vi "Delete Header Content Object.vi"(8 "error in (no error)":errorcluster, 11 "Header in":refnum<class "Simulated_Header.lvclass">) -> (0 "error out":errorcluster, 3 "Header out":refnum<class "Simulated_Header.lvclass">)   [LabVIEW 2018, in "Simulated_Header.lvclass"]
uses:
  Simulated_Header.lvclass
  Header Contents/Header Contents.lvclass
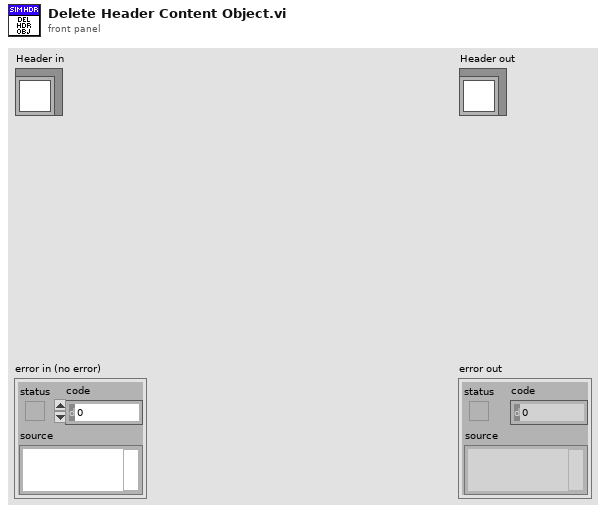
[diagram p1: front panel]
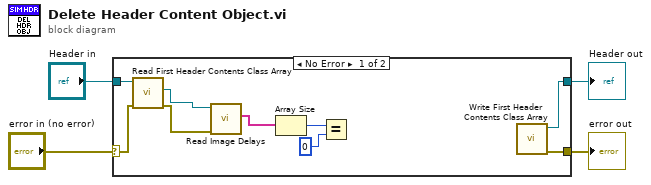
[diagram p0: block diagram]
diagram:
  n1 = case shown="No Error" "error in (no error)" {
    selector: "error in (no error)" -> [w11 w15]
    tunnel: [w12 w15] -> w3
    tunnel: [w13 w14] -> w1
    tunnel: "Header in" -> [w5 w14]
    frame No Error {
      n2 = call "Read First Header Contents Class Array .vi"("error in (no error)"=w11, "Simulated_Header in"=w5) -> ("error out"=w9:errorcluster, "Header Contents.lvclass"=w10:refnum<class "Header Contents.lvclass">)  [unwired: 7 in, 1 out]
      n3 = call "Read Image Delays.vi"("error in (no error)"=w9, "Header Contents in"=w10) -> ("Image Delays"=w8:string[])  [unwired: 7 in, 2 out]
      n4 = Array Size(array=w8) -> (size(s)=w7:i32)
      n5 = Equal?(x=w7, y=0) -> ()  [unwired: 1 out]
      n6 = call "Write First Header Contents Class Array .vi"() -> ("error out"=w12:errorcluster, "Simulated_Header out"=w13:refnum<class "Simulated_Header.lvclass">)  [unwired: 10 in]
    }
    frame Error {
    }
  }
  "error out" <- w3
  "Header out" <- w1
